vi "Load Test Executive.vi"(6 "Folder":path, 7 "Persistence in":refnum<class "IPersist.lvclass">, 8 "error in (no error)":errorcluster, 9 "Compatibility Helper":refnum<class "ICompatibility Helper.lvclass">, 10 "Path Builder":refnum<class "IPath Builder.lvclass">, 11 "Test Executive":refnum<class "ITest Executive.lvclass">) -> (0 "error out":errorcluster, 3 "Test Executive Ref out":refnum<data-value>, 5 "Root ID":string)   [LabVIEW 2017, in "Test Executive.lvlib" / "TestExecutive Ref.lvclass"]
uses:
  <vilib>/gpm_packages/@cs/test-executive/Source/Test Executive/TestExecutive Ref/TestExecutive Ref.lvclass
  <vilib>/gpm_packages/@cs/test-executive/Source/Test Executive/ITestExecutive/ITest Executive.lvclass
  <vilib>/gpm_packages/@cs/persistence/source/IPersist/IPersist.lvclass
  <vilib>/gpm_packages/@cs/test-executive/Source/Path Builder/IPath Builder/IPath Builder.lvclass
  <vilib>/gpm_packages/@cs/test-executive/Source/Compatibility Helper/ICompatibility Helper.lvclass
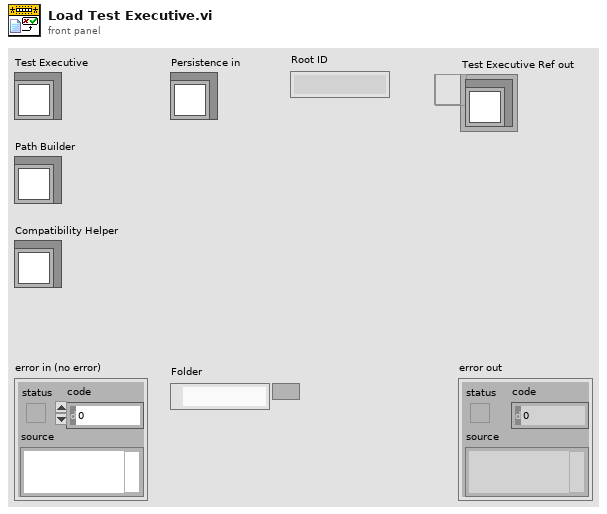
[diagram p1: front panel]
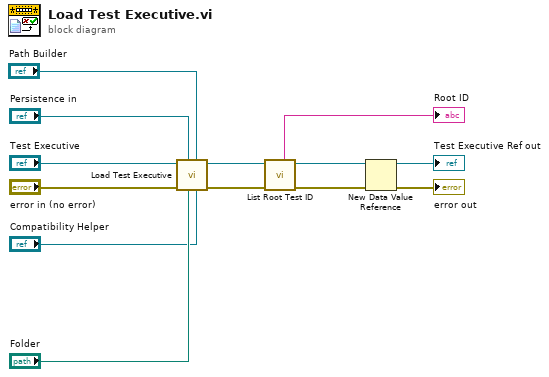
[diagram p0: block diagram]
diagram:
  n1 = call-dynamic "Load Test Executive.vi"("Compatibility Helper"="Compatibility Helper", "Path Builder"="Path Builder", "File Path"="Folder", "Persistence in"="Persistence in", "error in (no error)"="error in (no error)", "ITest Executive in"="Test Executive") -> ("error out"=w5:errorcluster, "ITest Executive out"=w7:refnum<class "ITest Executive.lvclass">)  [unwired: 4 in]
  n2 = call-dynamic "List Root Test ID.vi"("error in (no error)"=w5, "ITest Executive in"=w7) -> ("error out"=w4:errorcluster, "ITest Executive out"=w6:refnum<class "ITest Executive.lvclass">, "Root ID"=→"Root ID":string)  [unwired: 5 in, 2 out]
  n3 = New Data Value Reference(data value=w6, error in=w4) -> (data value reference=→"Test Executive Ref out":refnum<data-value>, error out=→"error out":errorcluster)
